vi "GetAllLibraries.vi"(8 "error in (no error)":errorcluster) -> (0 "error out":errorcluster, 3 "Lvlib paths":path[](array[path]))   [LabVIEW 2019, in "Hawkeye.lvlib"]
uses:
  Hawkeye.lvlib
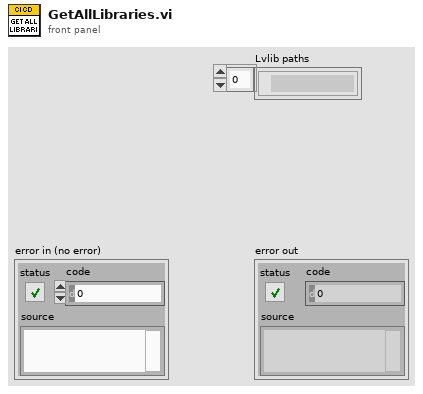
[diagram p1: front panel]
types:
  T1 = typedef "Hawkeye.lvlib/CICDPathConfigs.ctl" = cluster{"GlobalIncludePaths":path[], "GlobalExcludePaths":path[], "BuildSpecsIncludePaths":path[], "ActualDepsIncludePaths":path[], "WorkspacePath":path, "SourceFolderPaths":path[], "ChangedFilesLogpaths":map{string, path}}
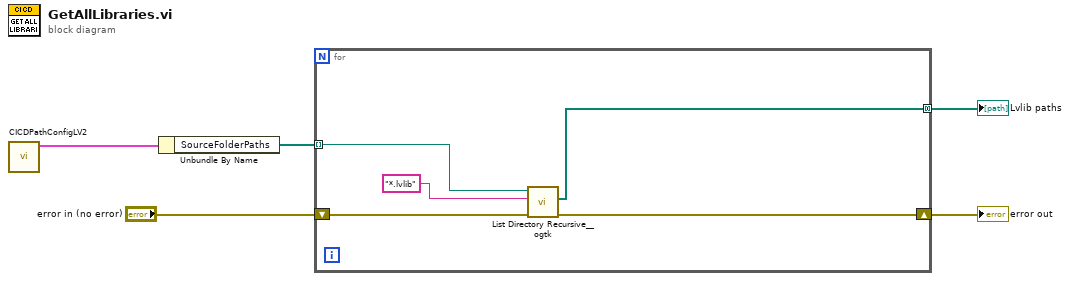
[diagram p0: block diagram]
diagram:
  n1 = call "CICDPathConfigLV2.vi"() -> ("CICD Path Config Out"=w1:T1)  [unwired: 11 in]
  n2 = Unbundle By Name(w1) -> ("SourceFolderPaths"=w4:path[])
  n3 = for {
    tunnel: [w6] -> w2 mode=concatenating
    shift-right: [w7] -> w3
    shift-left: "error in (no error)" -> [w10]
    tunnel: w4 -> [w8] mode=indexing
    n4 = call <userlib>:"List Directory Recursive__ogtk.vi"("error in (no error)"=w10, "pattern"="*.lvlib", "Path"=w8) -> ("error out"=w7:errorcluster, "file paths"=w6:path[])  [unwired: 5 in, 2 out]
  }
  "error out" <- w3
  "Lvlib paths" <- w2
